vi "Update Current Task Name.vi"(8 "error in (no error)":errorcluster, 10 "CurrentTaskName":string, 11 "BuildWorker in":refnum<class "BuildWorker.lvclass">) -> (0 "error out":errorcluster, 3 "BuildWorker out":refnum<class "BuildWorker.lvclass">)   [LabVIEW 2017, in "BuildWorker.lvlib" / "BuildWorker.lvclass"]
uses:
  BuildWorker.lvclass
  Classes/Task/Status.ctl
  Classes/Task/Task.lvclass
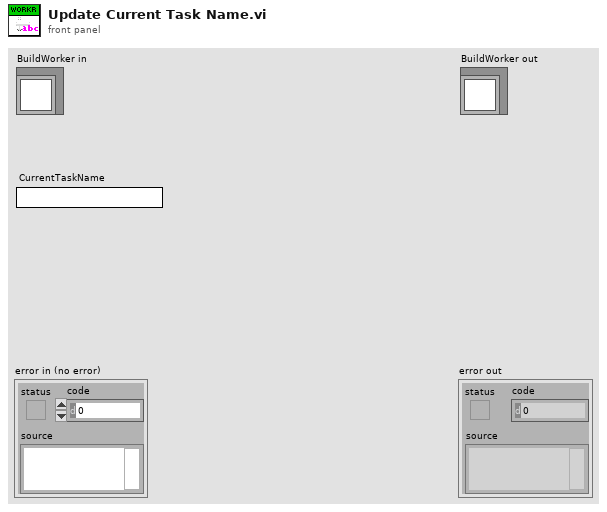
[diagram p1: front panel]
types:
  T1 = typedef "Task Interface.lvlib/Task.lvclass/Status.ctl" = enum16{"Created", "Added", "Pending", "Queued", "Processing", "Cleaning", "Building", "Finished", "Failed", "Removed", "Not found"}
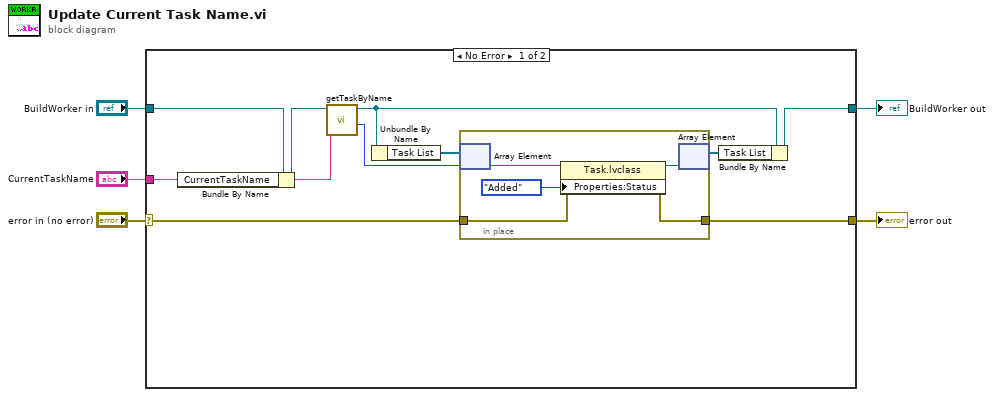
[diagram p0: block diagram]
diagram:
  n1 = case shown="No Error" "error in (no error)" {
    selector: "error in (no error)" -> [w7 w22]
    tunnel: [w6 w22] -> w4
    tunnel: [w9 w21] -> w2
    tunnel: "BuildWorker in" -> [w15 w21]
    tunnel: "CurrentTaskName" -> [w13 _]
    frame No Error {
      n2 = Bundle By Name(cluster=w15, "CurrentTaskName"=w13) -> (w14:refnum<class "BuildWorker.lvclass">)
      n3 = call "getTaskByName.vi"("Task Name"=w13, "BuildWorker in"=w14) -> ("index of element"=w10:i32, "BuildWorker out"=w12:refnum<class "BuildWorker.lvclass">)  [unwired: 7 in, 1 out]
      n4 = Unbundle By Name(w12) -> ("Task List"=w11:refnum<class "Task.lvclass">[])
      n5 = in-place {
        in-place-border: w7 -> [w16]
        in-place-border: [w17] -> w6
        n6 = in-place-array #1(w11, w10) -> (w19:refnum<class "Task.lvclass">)
        n7 = property class="Task.lvclass"(reference=w19, error in=w16, "Properties:Status"=Status."Added" ("Status")) -> (reference out=w18:refnum<class "Task.lvclass">, error out=w17:errorcluster)
        n8 = in-place-array #1(w18) -> (w8:refnum<class "Task.lvclass">[])  [unwired: 1 out]
      }
      n9 = Bundle By Name(cluster=w12, "Task List"=w8) -> (w9:refnum<class "BuildWorker.lvclass">)
    }
    frame Error {
    }
  }
  "error out" <- w4
  "BuildWorker out" <- w2
